vi "runDO_img.vi"   [LabVIEW 2015]
uses:
  waveforms/usedDOindepofwf.vi
  Objects/2pparameters.vi
  Objects/configuration.vi
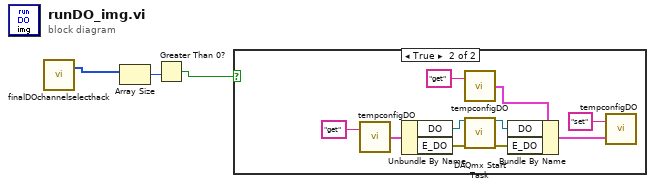
[diagram p0: block diagram]
diagram:
  n1 = call "finalDOchannelselecthack.vi"() -> ("usedDO"=w1:u32[])  [unwired: 1 in, 1 out]
  n2 = Array Size(array=w1) -> (size(s)=w3:i32)
  n3 = Greater Than 0?(x=w3) -> (x > 0?=w2:bool)
  n4 = case shown="True" w2 {
    frame False {
    }
    frame True {
      n5 = call "tempconfigDO.vi"("command"="get") -> ("Temp Config out"=w10:cluster{"DO":refnum<k21>, "E_DO":errorcluster})  [unwired: 1 in]
      n6 = Unbundle By Name(w10) -> ("DO"=w9:refnum<k21>, "E_DO"=w8:errorcluster)
      n7 = call "tempconfigDO.vi"("command"="get") -> ("Temp Config out"=w7:cluster{"DO":refnum<k21>, "E_DO":errorcluster})  [unwired: 1 in]
      n8 = call <vilib>:"DAQmx Start Task.vi"("task/channels in"=w9, "error in"=w8) -> ("task out"=w6:refnum<k21>, "error out"=w5:errorcluster)  [unwired: 12 in]
      n9 = Bundle By Name(cluster=w7, "DO"=w6, "E_DO"=w5) -> (w4:cluster{"DO":refnum<k21>, "E_DO":errorcluster})
      n10 = call "tempconfigDO.vi"("Temp Config in"=w4, "command"="set") -> ()  [unwired: 1 out]
    }
  }
